vi "Configure Measurment Mode.vi"(7 "Measurement 2 (0: thdAmplitude)":i32(ring) items=["thdAmplitude", "thdRatio"], 8 "error in (no error)":errorcluster, 9 "Measurement 1 (0: thdAmplitude)":i32(ring) items=["thdAmplitude", "thdRatio"], 10 "Analyzer (0: A0)":i32(ring) items=["A0", "A1"], 11 "VISA resource name":refnum<visa-resource-name>) -> (0 "error out":errorcluster, 3 "VISA resource name out":refnum<visa-resource-name>)   [LabVIEW 2014, in "Stanford Research SR1.lvlib"]
doc: "Configures the attributes for the Measurement Mode."
uses:
  Stanford Research SR1.lvlib
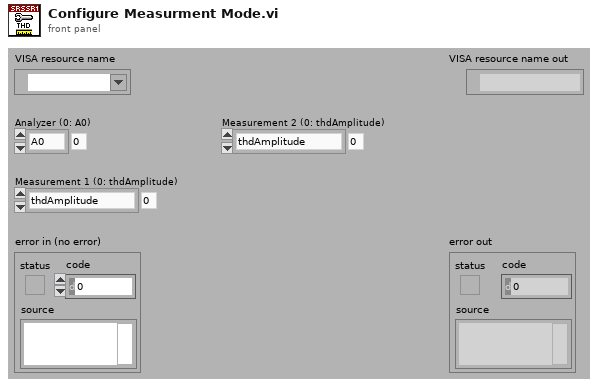
[diagram p1: front panel]
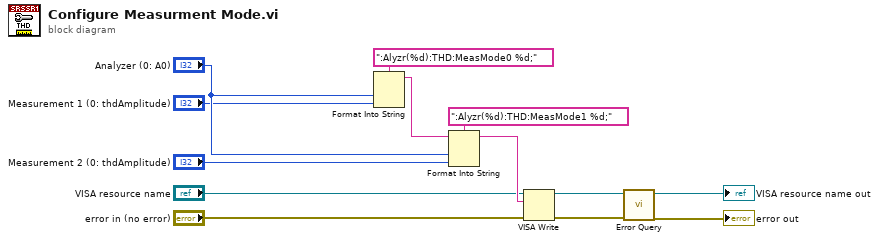
[diagram p0: block diagram]
diagram:
  n1 = Format Into String(format string=":Alyzr(%d):THD:MeasMode0 %d;", "Analyzer (0: A0)", "Measurement 1 (0: thdAmplitude)") -> (resulting string=w12:string)  [unwired: 2 in, 1 out]
  n2 = Format Into String(format string=":Alyzr(%d):THD:MeasMode1 %d;", initial string=w12, "Analyzer (0: A0)", "Measurement 2 (0: thdAmplitude)") -> (resulting string=w10:string)  [unwired: 1 in, 1 out]
  n3 = VISA Write(VISA resource name="VISA resource name", write buffer=w10, error in (no error)="error in (no error)") -> (VISA resource name out=w7:refnum<visa-resource-name>, error out=w6:errorcluster)  [unwired: 1 out]
  n4 = call "Error Query.vi"("error in (no error)"=w6, "VISA resource name"=w7) -> ("error out"=→"error out":errorcluster, "VISA resource name out"=→"VISA resource name out":refnum<visa-resource-name>)  [unwired: 6 in, 2 out]
